vi "Byte To SDIR.vi"(11 "Numeric":u8) -> (3 "DIR":T1)   [LabVIEW 2022 SP3, in "FHPP.lvclass"]
uses:
  FHPP.lvclass
  FHPP.lvclass/FHPP.ctl
  TypeDefs/DIR.ctl
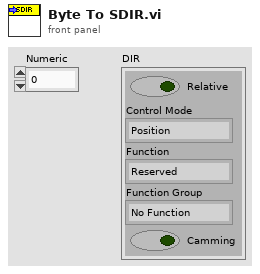
[diagram p1: front panel]
types:
  T1 = typedef "FHPP.lvclass/DIR.ctl" = cluster{"Relative":bool, "Control Mode":enum8{"Position", "Force", "Velocity", "Reserved"}, "Function":enum8{"Reserved", "External Input", "External Input with  Cam", "Virtual Master with Cam"}, "Function Group":enum8{"No Function", "Reserver 1", "Reserved 2", "Reserved 3"}, "Camming":bool}
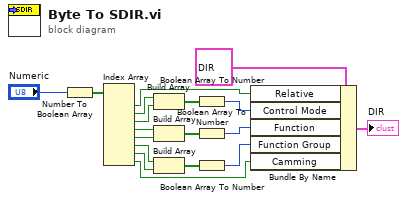
[diagram p0: block diagram]
diagram:
  n1 = Number To Boolean Array(number="Numeric") -> (Boolean array=w16:bool[])
  n2 = Index Array(array=w16) -> (element #1=w15:bool, element #2=w14:bool, element #3=w13:bool, element #4=w8:bool, element #5=w7:bool, element #6=w6:bool, element #7=w5:bool, element #8=w2:bool)  [unwired: 8 in]
  n3 = Build Array(w14, w13) -> (w12:bool[])
  n4 = Build Array(w8, w7) -> (w10:bool[])
  n5 = Build Array(w6, w5) -> (w9:bool[])
  n6 = Boolean Array To Number(Boolean array=w12) -> (number=w11:u8)
  n7 = Boolean Array To Number(Boolean array=w10) -> (number=w4:u8)
  n8 = Boolean Array To Number(Boolean array=w9) -> (number=w3:u8)
  n9 = Bundle By Name(cluster=T1 {"Relative"=FALSE, "Control Mode"=enum."Position", "Function"=enum."Reserved", "Function Group"=enum."No Function", "Camming"=FALSE} ("DIR"), "Relative"=w15, "Control Mode"=w11, "Function"=w4, "Function Group"=w3, "Camming"=w2) -> (→"DIR":T1)
